vi "Simulate Self Test.vi"() -> (3 "Result":bool)   [LabVIEW 2015, in "Device Under Test_Cloneable_DQMH.lvlib"]
doc: "Generate a simulated self test result.\n____\nDelacor QMH Thermal Chamber Examples 4.0.0.21\nCopyright (c) 2018, Delacor"
uses:
  Device Under Test_Cloneable_DQMH.lvlib
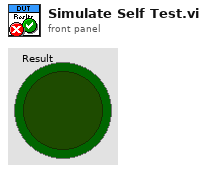
[diagram p1: front panel]
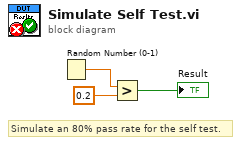
[diagram p0: block diagram]
diagram:
  # "Simulate an 80% pass rate for the self test."
  n1 = Random Number (0-1)() -> (number: 0 to 1=w1:dbl)
  n2 = Greater?(x=w1, y=0.2) -> (0:→"Result":bool)
